vi "Aktualizacja położenia i azymutu robota po kinematyce.vi"(6 "Aktualne położenie":T1, 8 "Rzeczywista odległość robota od startu [m]":cluster{"X [m]":dbl, "Y [m]":dbl}, 9 "Punkt docelowy":u16, 10 "Lista współrzędnych":string[][](array[string]), 11 "Boolean in":refnum<vi>) -> (0 "Odległość robota od startu":cluster{"X[m]":dbl, "Y[m]":dbl}, 1 "Zmiana położenia robota?":bool, 2 "Odl. robota od startu po kin.":dbl, 3 "Prędkości kół":T2, 4 "Aktualne położenie  2":T1)   [LabVIEW 2015, in "Biblioteka moduł map v3.lvlib" / "Pomocnicze.lvlib"]
uses:
  Pomocnicze.lvlib
  Matematyczne/Matematyczne.lvlib
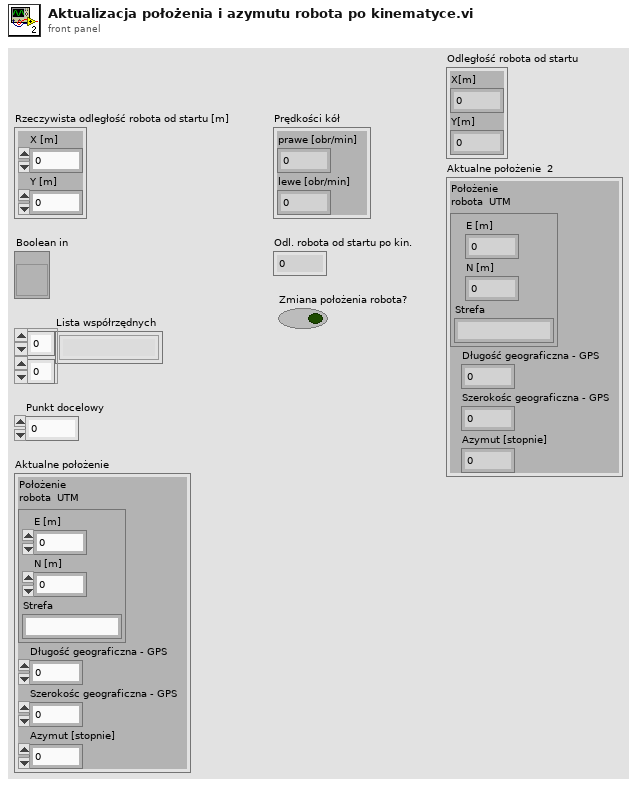
[diagram p1: front panel]
types:
  T1 = cluster{"Położenie \nrobota  UTM":cluster{"E [m]":ext, "N [m]":ext, "Strefa":string}, "Długość geograficzna - GPS":dbl, "Szerokośc geograficzna - GPS":dbl, "Azymut [stopnie]":dbl}
  T2 = cluster{"prawe [obr/min]":dbl, "lewe [obr/min]":dbl}
  T3 = cluster{"prawe [obr/min]":i64, "lewe [obr/min]":i64}
  T4 = cluster{"Promień koła [m]":dbl, "Szerokość robota [m]":dbl}
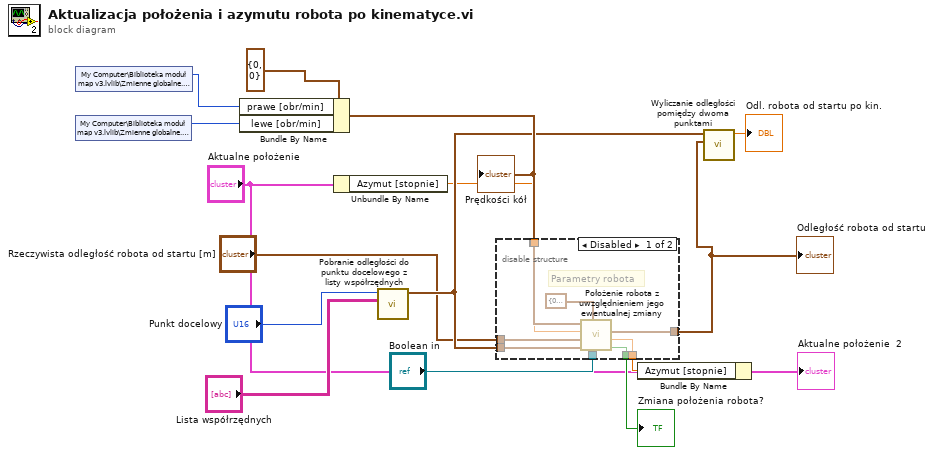
[diagram p0: block diagram]
diagram:
  n1 = shared-variable "My Computer\\Biblioteka moduł map v3.lvlib\\Zmienne globalne.lvlib\\Vr obr na min"() -> (w5:i64)  [unwired: 1 in, 1 out]
  n2 = shared-variable "My Computer\\Biblioteka moduł map v3.lvlib\\Zmienne globalne.lvlib\\Vl obr na min"() -> (w4:i64)  [unwired: 1 in, 1 out]
  n3 = Bundle By Name(cluster=T3 {"prawe [obr/min]"=0, "lewe [obr/min]"=0} ("Prędkości kół"), "prawe [obr/min]"=w5, "lewe [obr/min]"=w4) -> (w15:T3)
  "Prędkości kół" <- w15
  n4 = Unbundle By Name("Aktualne położenie") -> ("Azymut [stopnie]"=w8:dbl)
  n5 = call "Pobranie odległości do punktu docelowego z listy współrzędnych.vi"("Lista współrzędnych"="Lista współrzędnych", "Numer pobranego punktu"="Punkt docelowy") -> ("Odl. pkt. od bazy"=w14:cluster{"E/x[m]":dbl, "N/y[m]":dbl})  [unwired: 6 in, 3 out]
  n6 = disable-structure shown="Disabled" {
    disable-tunnel: [w25 _] -> w16
    disable-tunnel: w15 -> [w24 _]
    disable-tunnel: w14 -> [w23 _]
    disable-tunnel: "Rzeczywista odległość robota od startu [m]" -> [w22 w26]
    disable-tunnel: [w21 w26] -> w9
    disable-tunnel: w8 -> [w20 _]
    disable-tunnel: [w19 _] -> w7
    disable-tunnel: "Boolean in" -> [w18 _]
    frame Disabled {
      # "Parametry robota"
      n7 = call "Położenie robota z uwzględnieniem jego ewentualnej zmiany.vi"("Zmiana poł. na mapie"=w18, "Parametry robota"=T4 {"Promień koła [m]"=0.045, "Szerokość robota [m]"=0.37}, "Odległość punktu\n docelowego od startu [m]"=w23, "Nowa Odl. od startu[m]"=w22, "Azymut robota pocz./nowy"=w20, "Prędkości kół"=w24) -> ("Zmiana położenia robota?"=w25:bool, "Azymut [stopnie]"=w19:dbl, "Odległość robota od startu"=w21:cluster{"X[m]":dbl, "Y[m]":dbl})  [unwired: 3 in]
    }
    frame Enabled {
    }
  }
  "Zmiana położenia robota?" <- w16
  "Odległość robota od startu" <- w9
  n8 = Bundle By Name(cluster="Aktualne położenie", "Azymut [stopnie]"=w7) -> (→"Aktualne położenie  2":T1)
  n9 = call "Wyliczanie odległości pomiędzy dwoma punktami.vi"("Polozenie 1"=w9, "Polozenie in"=w14) -> ("Numeric"=→"Odl. robota od startu po kin.":dbl)  [unwired: 9 in]
